vi "Untitled 3.vi"() -> ()   [LabVIEW 2018]
panel:
  out "Output":dbl
  in  "2nd number":dbl
  in  "1st number":dbl
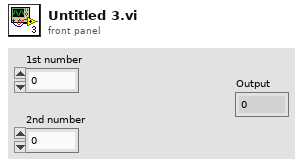
[diagram p1: front panel]
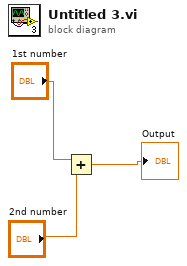
[diagram p0: block diagram]
diagram:
  n1 = Add(x="1st number", y="2nd number") -> (x+y=→"Output":dbl)
